vi "Test_target.vi"() -> ()   [LabVIEW 2013]
uses:
  <vilib>/rvi/Emulation/niFpgaSctlEmulationGetInTimedLoop.vi
  <vilib>/rvi/Emulation/niFpgaEmulationReportErrorSimple.vi
  <vilib>/rvi/eio/common/nirviEmuTemplateMethod_errors.vi
  <vilib>/rvi/Emulation/niFpgaGetClockAttributes.vi
  <vilib>/rvi/Emulation/niFpgaCriticalErrorInLSC.vi
  <vilib>/eio/EIONode/EIONode.xnode
panel:
  in  "Boolean":bool=TRUE
  in  "stop":bool
  in  "WRITE":bool=TRUE
  in  "WE2":bool
  in  "WE1":bool=TRUE
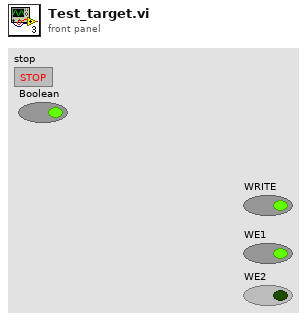
[diagram p1: front panel]
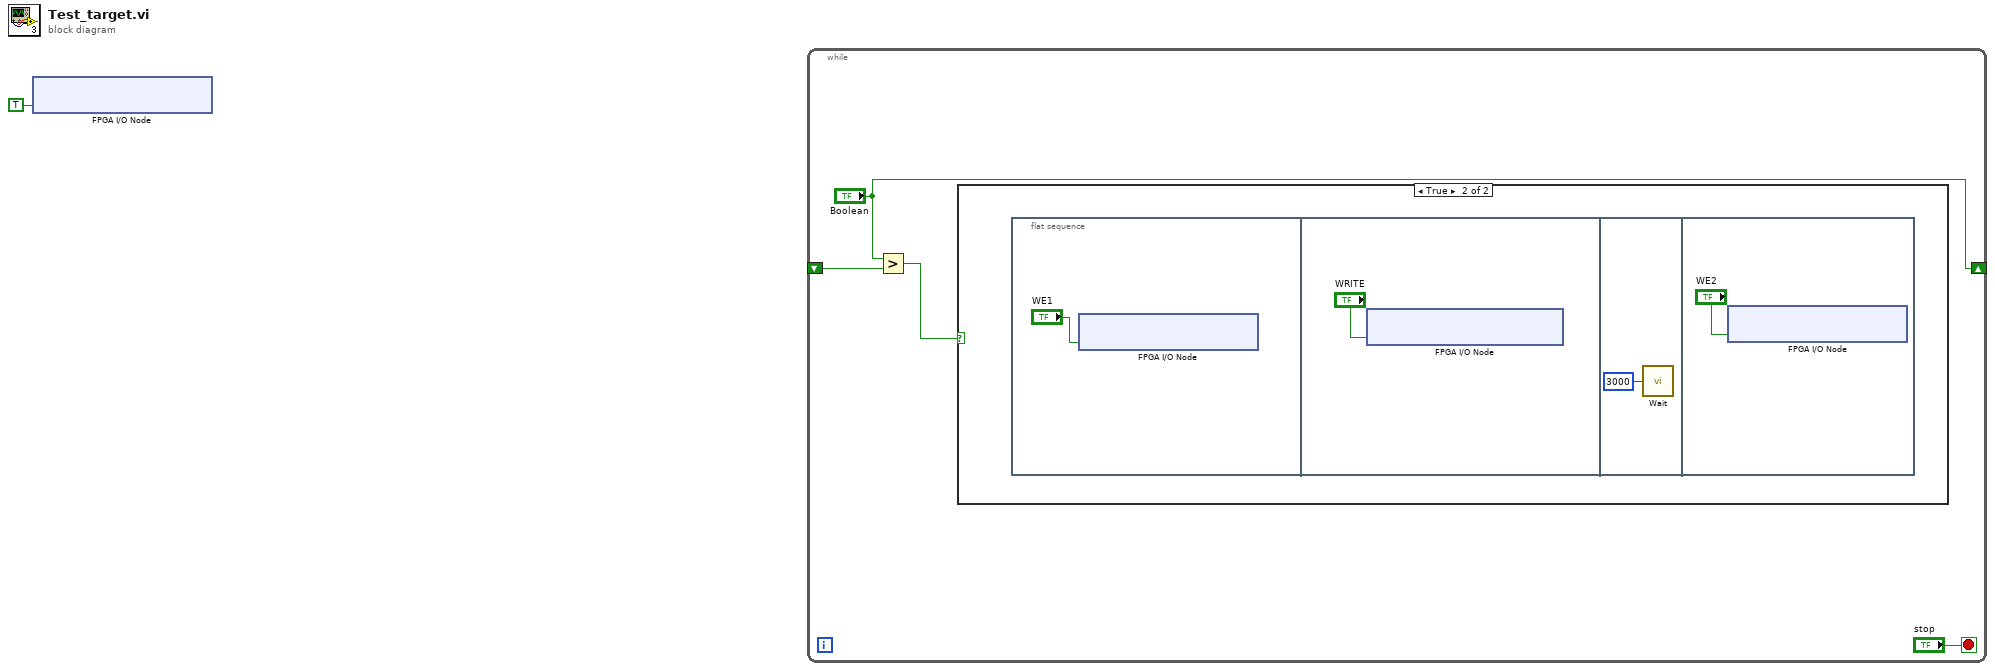
[diagram p0: block diagram]
diagram:
  n1 = xnode "FPGA I/O Node"("IO Module\\DDCA_PFI_WE"=TRUE ("IO Module\\DDCA_DIO0-7_WE")) -> ()  [unwired: 1 in, 1 out]
  n2 = while {
    shift-right: ["Boolean"] -> _
    shift-left: _ -> [w4]
    stop <- "stop" stop-if-true
    n3 = Greater?(x="Boolean", y=w4) -> (0:w2:bool)
    n4 = case shown="True" w2 {
      frame False {
      }
      frame True {
        n5 = flat-sequence {
          frame #0 {
            n6 = xnode "FPGA I/O Node"("IO Module\\DDCA_PFI_WE"="WE1") -> ()  [unwired: 1 in, 1 out]
          }
          frame #1 {
            n7 = xnode "FPGA I/O Node"("IO Module\\DDCA_PFI1_Write"="WRITE") -> ()  [unwired: 1 in, 1 out]
          }
          frame #2 {
            n8 = call "Wait"("Count(mSec)"=u32 3000) -> ()  [unwired: 1 out]
          }
          frame #3 {
            n9 = xnode "FPGA I/O Node"("IO Module\\DDCA_PFI_WE"="WE2") -> ()  [unwired: 1 in, 1 out]
          }
        }
      }
    }
  }
